vi "PrepareForVision.vi"(10 "CameraVideoMode":u32, 11 "InterfaceName":string) -> (0 "error out":errorcluster, 1 "DisplayImageRef":T2, 2 "VisionImageRef":T2, 3 "CameraSessionOut":T1)   [LabVIEW 2017]
uses:
  <vilib>/vision/Image Controls.llb/IMAQ Image.ctl
  <vilib>/userdefined/High Color/IMAQdx.ctl
  <vilib>/vision/driver/IMAQdx.llb/IMAQdx Camera Control Mode.ctl
  <vilib>/vision/driver/NI_Vision_Acquisition_Software.lvlib
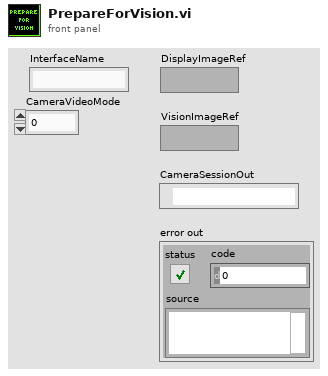
[diagram p1: front panel]
types:
  T1 = typedef "IMAQdx.ctl" = refnum<k21>
  T2 = typedef "IMAQ Image.ctl" = refnum<image>
  T3 = typedef "Image Type" = u32
  T4 = typedef "NI_Vision_Acquisition_Software.lvlib/IMAQdx Camera Control Mode.ctl" = enum32{"Controller", "Listener"}
  T5 = cluster{"Type":u32, "Version":u32, "Flags":u32, "SerialNumberHigh":u32, "SerialNumberLow":u32, "BusType":u32, "InterfaceName":string, "VendorName":string, "ModelName":string, "CameraFileName":string, "CameraAttributeURL":string}[]
  T6 = cluster{"Type":u32, "Version":u32, "Flags":u32, "SerialNumberHigh":u32, "SerialNumberLow":u32, "BusType":u32, "InterfaceName":string, "VendorName":string, "ModelName":string, "CameraFileName":string, "CameraAttributeURL":string}
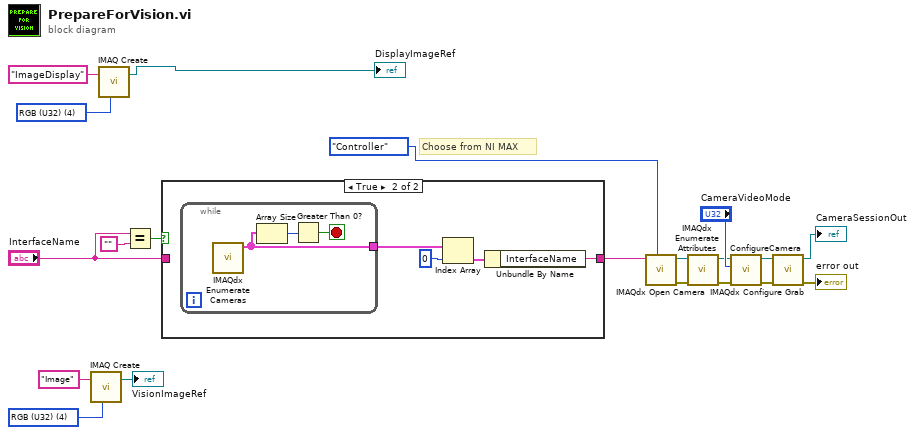
[diagram p0: block diagram]
diagram:
  w17 = T3 4 items=["Grayscale (U8)", "Grayscale (I16)", "Grayscale (SGL)", "Complex (CSG)", "RGB (U32)", "HSL (U32)", "RGB (U64)", "Grayscale (U16)"] ("Image Type")
  w12 = T3 4 items=["Grayscale (U8)", "Grayscale (I16)", "Grayscale (SGL)", "Complex (CSG)", "RGB (U32)", "HSL (U32)", "RGB (U64)", "Grayscale (U16)"] ("Image Type")
  # "Choose from NI MAX"
  n1 = call "IMAQ Create"("Image Name"="Image", "Image Type"=w12) -> ("New Image"=→"VisionImageRef":T2)  [unwired: 3 in, 1 out]
  n2 = call "IMAQ Create"("Image Name"="ImageDisplay", "Image Type"=w17) -> ("New Image"=→"DisplayImageRef":T2)  [unwired: 3 in, 1 out]
  n3 = Equal?(x="InterfaceName", y="") -> (x = y?=w19:bool)
  n4 = case shown="True" w19 {
    tunnel: [w21 w22] -> w2
    tunnel: "InterfaceName" -> [w21 _]
    frame False {
    }
    frame True {
      n5 = while {
        tunnel: [w26] -> w25
        stop <- w27 stop-if-true
        n6 = call <vilib>:"IMAQdx Enumerate Cameras.vi"() -> ("Camera Information Array"=w26:T5)  [unwired: 10 in, 1 out]
        n7 = Array Size(array=w26) -> (size(s)=w28:i32)
        n8 = Greater Than 0?(x=w28) -> (x > 0?=w27:bool)
      }
      n9 = Index Array(array=w25, index=0) -> (element=w23:T6)
      n10 = Unbundle By Name(w23) -> ("InterfaceName"=w22:string)
    }
  }
  n11 = call <vilib>:"IMAQdx Open Camera.vi"("Camera Control Mode"=IMAQdx_Camera_Control_Mode."Controller", "Session In"=w2) -> ("error out"=w4:errorcluster, "Session Out"=w5:T1)  [unwired: 8 in]
  n12 = call <vilib>:"IMAQdx Enumerate Attributes.vi"("error in"=w4, "Session In"=w5) -> ("error out"=w7:errorcluster, "Session Out"=w6:T1)  [unwired: 7 in, 1 out]
  n13 = call "ConfigureCamera.vi"("error in (no error)"=w7, "CameraVideoMode"="CameraVideoMode", "Refnum in"=w6) -> ("error out"=w10:errorcluster, "Refnum out"=w9:T1)  [unwired: 7 in]
  n14 = call <vilib>:"IMAQdx Configure Grab.vi"("error in"=w10, "Session In"=w9) -> ("error out"=→"error out":errorcluster, "Session Out"=→"CameraSessionOut":T1)  [unwired: 8 in]
